vi "Get IC.vi"(8 "error in (no error)":errorcluster, 10 "Domain":refnum<class "NI_Domain.lvclass">, 11 "IC_1D_VIRef in":refnum<class "NI_IC_1D_VIRef.lvclass">) -> (0 "error out":errorcluster, 2 "IC":variant, 3 "IC_1D_VIRef out":refnum<class "NI_IC_1D_VIRef.lvclass">)   [LabVIEW 2017, in "NI_PDE.lvlib" / "NI_IC_1D_VIRef.lvclass"]
uses:
  <vilib>/gmath/pde.llb/ICClass/IC_1D_VIRef/NI_IC_1D_VIRef.lvclass
  <vilib>/gmath/pde.llb/DomainClass/NI_Domain.lvclass
  <vilib>/gmath/pde.llb/ICClass/IC_1D_VIRef/IC Data.ctl
  <vilib>/gmath/pde.llb/Common/PDE_IC Type.ctl
  <vilib>/gmath/pde.llb/ICClass/IC_1D_VIRef/NI_IC_1D_VIRef.lvclass/NI_IC_1D_VIRef.ctl
  <vilib>/gmath/NI_PDE.lvlib
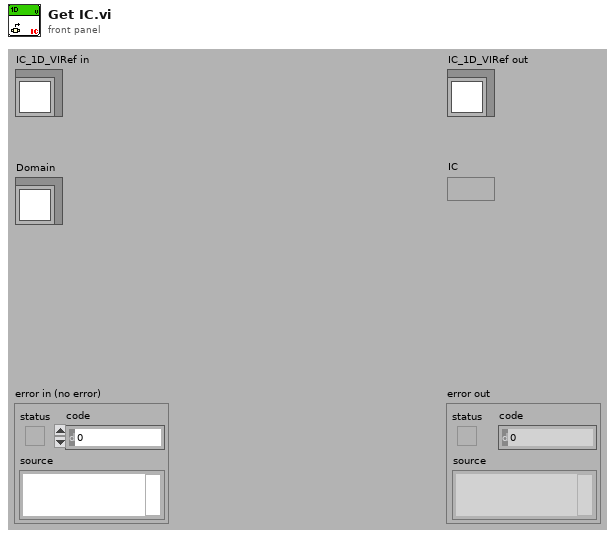
[diagram p1: front panel]
types:
  T1 = typedef "NI_PDE.lvlib/NI_IC_1D_VIRef.lvclass/IC Data.ctl" = cluster{"type":T2, "H":refnum<vi>, "data":variant}
  T2 = typedef "NI_PDE.lvlib/PDE_IC Type.ctl" = i32
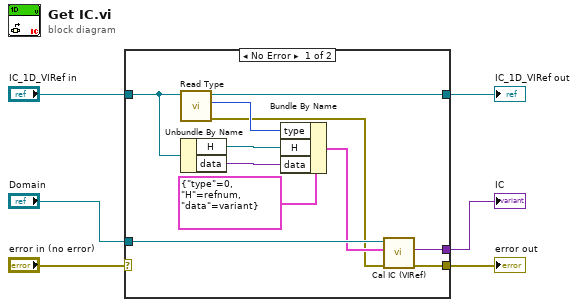
[diagram p0: block diagram]
diagram:
  n1 = case shown="No Error" "error in (no error)" {
    selector: "error in (no error)" -> [_ w18]
    tunnel: "IC_1D_VIRef in" -> [w14 w19]
    tunnel: [w9 _] -> w3
    tunnel: [w17 w19] -> w6
    tunnel: [w8 w18] -> w4
    tunnel: "Domain" -> [w11 _]
    frame No Error {
      n2 = call-dynamic "Read Type.vi"("IC.lvclass in"=w14) -> ("error out"=w7:errorcluster, "IC type"=w15:T2, "IC.lvclass out"=w17:refnum<class "NI_IC_1D_VIRef.lvclass">)  [unwired: 1 in, 7 out]
      n3 = Unbundle By Name(w14) -> ("H"=w13:refnum<vi>, "data"=w12:variant)
      n4 = Bundle By Name(cluster=T1 {"type"=0, "H"=refnum, "data"=variant} ("IC data"), "type"=w15, "H"=w13, "data"=w12) -> (w10:T1)
      n5 = call-dynamic "Cal IC (VIRef).vi"("error in (no error)"=w7, "IC in"=w10, "Domain in"=w11) -> ("error out"=w8:errorcluster, "IC out"=w9:variant)  [unwired: 7 out]
    }
    frame Error {
    }
  }
  "IC" <- w3
  "error out" <- w4
  "IC_1D_VIRef out" <- w6
